vi "Total Obst Detection HC-SR04 Module.vi"(0 "FPGA VI Reference In":refnum<k20>, 7 "Threshold":sgl=2.3, 11 "Error In":errorcluster) -> (1 "US FR":sgl, 2 "US FL":sgl, 3 "US BK":sgl, 4 "FPGA VI Reference Out":refnum<k20>, 12 "US FR":bool, 13 "US FL":bool, 14 "US BK":bool, 15 "Error Out":errorcluster)   [LabVIEW 2015]
panel:
  out "Accelerometer":cluster{"Z":i16, "Y":i16, "X":i16}
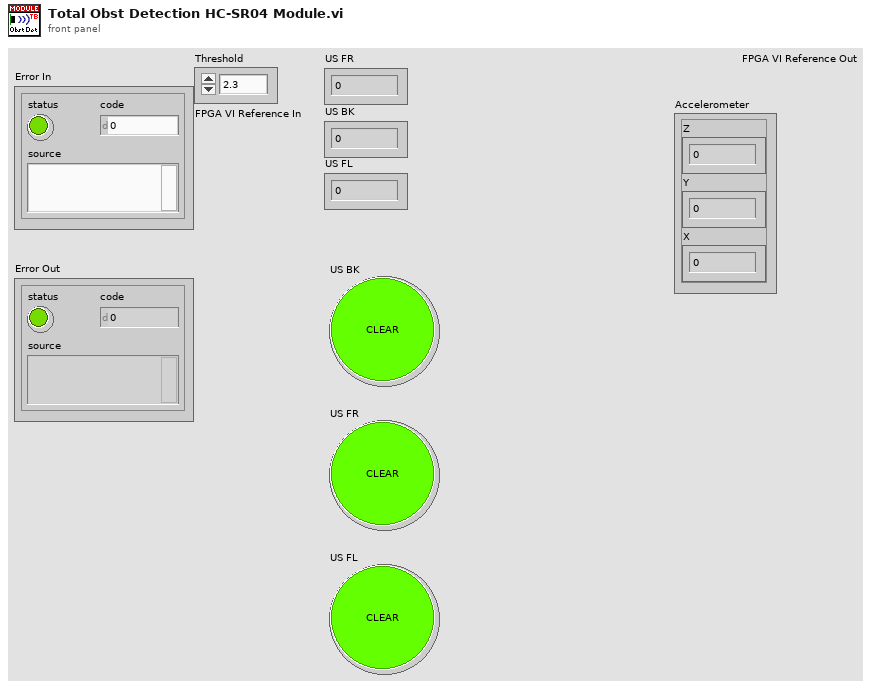
[diagram p1: front panel]
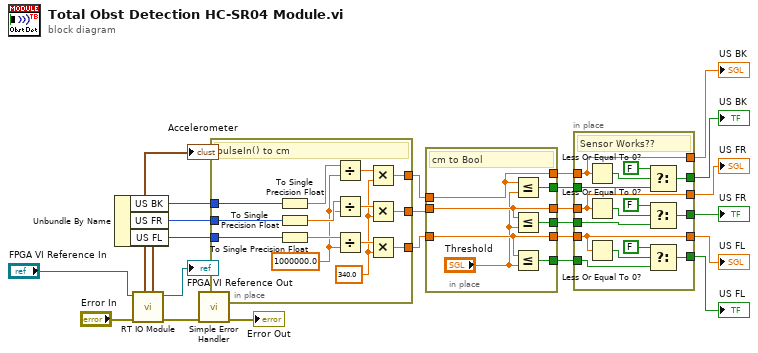
[diagram p0: block diagram]
diagram:
  n1 = call "RT IO Module.vi"("FPGA VI Reference In"="FPGA VI Reference In", "Error In"="Error In") -> ("Accelerometer"=→"Accelerometer":cluster{"Z":i16, "Y":i16, "X":i16}, "Ultrasuond"=w22:cluster{"US BK":i16, "US FR":i16, "US FL":i16}, "FPGA VI Reference Out"=→"FPGA VI Reference Out":refnum<k20>, "Error Out"=w23:errorcluster)  [unwired: 2 in, 3 out]
  n2 = Unbundle By Name(w22) -> ("US BK"=w5:i16, "US FR"=w4:i16, "US FL"=w3:i16)
  n3 = call <vilib>:"Simple Error Handler.vi"("error in (no error)"=w23) -> ("error out"=→"Error Out":errorcluster)  [unwired: 4 in, 4 out]
  n4 = in-place {
    in-place-border: w5 -> [w39]
    in-place-border: w4 -> [w38]
    in-place-border: w3 -> [w37]
    in-place-border: [w28] -> w1
    in-place-border: [w27] -> w6
    in-place-border: [w26] -> w2
    w29 = sgl 340.0 ("y")
    w33 = sgl 1000000.0 ("y")
    # "pulseIn() to cm"
    n5 = To Single Precision Float(number=w39) -> (single precision float=w36:sgl)
    n6 = To Single Precision Float(number=w38) -> (single precision float=w35:sgl)
    n7 = To Single Precision Float(number=w37) -> (single precision float=w34:sgl)
    n8 = Divide(x=w36, y=w33) -> (x/y=w32:sgl)
    n9 = Divide(x=w35, y=w33) -> (x/y=w31:sgl)
    n10 = Divide(x=w34, y=w33) -> (x/y=w30:sgl)
    n11 = Multiply(x=w32, y=w29) -> (x*y=w26:sgl)
    n12 = Multiply(x=w31, y=w29) -> (x*y=w27:sgl)
    n13 = Multiply(x=w30, y=w29) -> (x*y=w28:sgl)
  }
  n14 = in-place {
    in-place-border: w1 -> [w41]
    in-place-border: w6 -> [w42]
    in-place-border: w2 -> [w43]
    in-place-border: [w46] -> w19
    in-place-border: [w45] -> w20
    in-place-border: [w44] -> w21
    in-place-border: [w43] -> w15
    in-place-border: [w42] -> w14
    in-place-border: [w41] -> w13
    # "cm to Bool"
    n15 = Less Or Equal?(x=w43, y="Threshold") -> (x <= y?=w46:bool)
    n16 = Less Or Equal?(x=w42, y="Threshold") -> (x <= y?=w45:bool)
    n17 = Less Or Equal?(x=w41, y="Threshold") -> (x <= y?=w44:bool)
  }
  n18 = in-place {
    in-place-border: w21 -> [w61]
    in-place-border: w20 -> [w60]
    in-place-border: w19 -> [w59]
    in-place-border: [w58] -> w18
    in-place-border: [w57] -> w17
    in-place-border: [w56] -> w16
    in-place-border: w15 -> [w49]
    in-place-border: w14 -> [w48]
    in-place-border: w13 -> [w47]
    in-place-border: [w49] -> w12
    in-place-border: [w48] -> w11
    in-place-border: [w47] -> w10
    # "Sensor Works??"
    n19 = Less Or Equal To 0?(x=w49) -> (x <= 0?=w52:bool)
    n20 = Less Or Equal To 0?(x=w48) -> (x <= 0?=w51:bool)
    n21 = Less Or Equal To 0?(x=w47) -> (x <= 0?=w50:bool)
    n22 = Select(t=FALSE, s=w52, f=w59) -> (s? t:f=w58:bool)
    n23 = Select(t=FALSE, s=w51, f=w60) -> (s? t:f=w57:bool)
    n24 = Select(t=FALSE, s=w50, f=w61) -> (s? t:f=w56:bool)
  }
  "US FR" <- w11
  "US BK" <- w12
  "US FL" <- w10
  "US BK" <- w18
  "US FR" <- w17
  "US FL" <- w16
